vi "Configure Integration Time.vi"(8 "error in (no error)":errorcluster, 10 "Integration Time (6000)":u32=6000, 11 "VISA resource name":refnum<visa-resource-name>) -> (0 "error out":errorcluster, 3 "VISA resource name out":refnum<visa-resource-name>)   [LabVIEW 2023, in "Ocean Optics 2000 4000.lvlib"]
doc: "Configures the integration time of the spectrometer. The integration time is the amount of time that the device collects light before digitizing it and sending it out over the USB. The longer the integration time, the more light it may collect."
uses:
  <instrlib>/Ocean Optics 2000 4000/Ocean Optics 2000 4000.lvlib
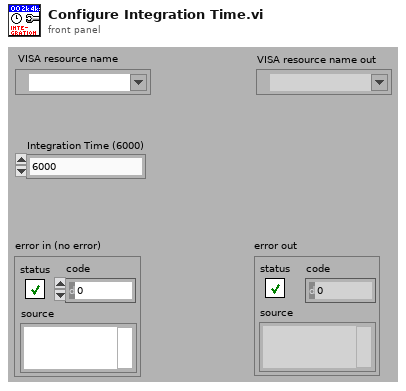
[diagram p1: front panel]
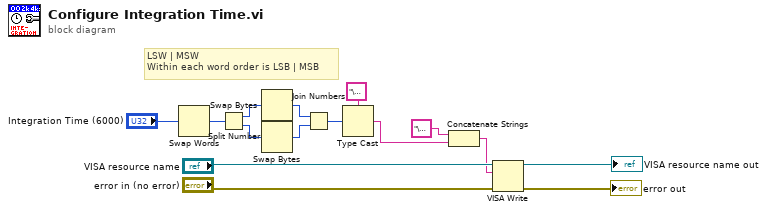
[diagram p0: block diagram]
diagram:
  # "LSW | MSW\nWithin each word order is LSB | MSB"
  n1 = Swap Words(1:"Integration Time (6000)") -> (0:w10:u32)
  n2 = Split Number(x=w10) -> (hi(x)=w9:u16, lo(x)=w8:u16)
  n3 = Swap Bytes(anything=w9) -> (byte swapped=w7:u16)
  n4 = Swap Bytes(anything=w8) -> (byte swapped=w6:u16)
  n5 = Join Numbers(hi=w7, lo=w6) -> ((hi.lo)=w5:u32)
  n6 = Type Cast(type="\u0000", x=w5) -> (*(type *) &x=w4:string)
  n7 = Concatenate Strings("\u0002" ("string"), w4) -> (w13:string)
  n8 = VISA Write(VISA resource name="VISA resource name", write buffer=w13, error in (no error)="error in (no error)") -> (VISA resource name out=→"VISA resource name out":refnum<visa-resource-name>, error out=→"error out":errorcluster)  [unwired: 1 out]
